vi "ProbePlanGenerator.vi"() -> ()   [LabVIEW 2013]
panel:
  in  "ATLAS 07 / ATLAS 12":u16(ring) items=["ATLAS 07", "ATLAS 12"]
  in  "innercut sensor?":bool
  in  "Filename":string="atlas12_innerc.txt"
  in  "Cancel Button":bool
  in  "Paste Button":bool
  in  "From 4-2":u16(ring) caption="From"
  in  "To 8":u16(ring) caption="To"
  in  "Column 4-2":u16(ring) caption="Column 2" items=["Column A", "Column B", "Column E", "Column C", "Column D"]
  in  "change4":bool caption="change columns?"
  in  "From 4-1":u16(ring) caption="From"
  in  "To 7":u16(ring) caption="To"
  in  "Column 4-1":u16(ring) caption="Column" items=["Column A", "Column B", "Column E", "Column C", "Column D"]
  in  "From 3-2":u16(ring) caption="From"
  in  "To 6":u16(ring) caption="To"
  in  "Column 3-2":u16(ring) caption="Column 2" items=["Column A", "Column B", "Column E", "Column C", "Column D"]
  in  "change3":bool caption="change columns?"
  in  "From 3-1":u16(ring) caption="From"
  in  "To 5":u16(ring) caption="To"
  in  "Column 3-1":u16(ring) caption="Column" items=["Column A", "Column B", "Column E", "Column C", "Column D"]
  in  "From 2-2":u16(ring) caption="From"
  in  "To 4":u16(ring) caption="To"
  in  "Column 2-2":u16(ring) caption="Column 2" items=["Column A", "Column B", "Column E", "Column C", "Column D"]
  in  "change2":bool caption="change columns?"
  in  "From 2-1":u16(ring) caption="From"
  in  "To 3":u16(ring) caption="To"
  in  "Column 2-1":u16(ring) caption="Column" items=["Column A", "Column B", "Column E", "Column C", "Column D"]
  in  "From 1-2":u16(ring) caption="From"
  in  "To 2":u16(ring) caption="To"
  in  "Column 1-2":u16(ring) caption="Column 2" items=["Column A", "Column B", "Column E", "Column C", "Column D"]
  in  "change1":bool caption="change columns?"
  in  "From 1-1":u16(ring) caption="From"
  in  "To":u16(ring)
  in  "Column 1-1":u16(ring) caption="Column" items=["Column A", "Column B", "Column E", "Column C", "Column D"]
  # "Probeplan Generator"
  # "Region 1"
  # "Region 2"
  # "Region 3"
  # "Region 4"
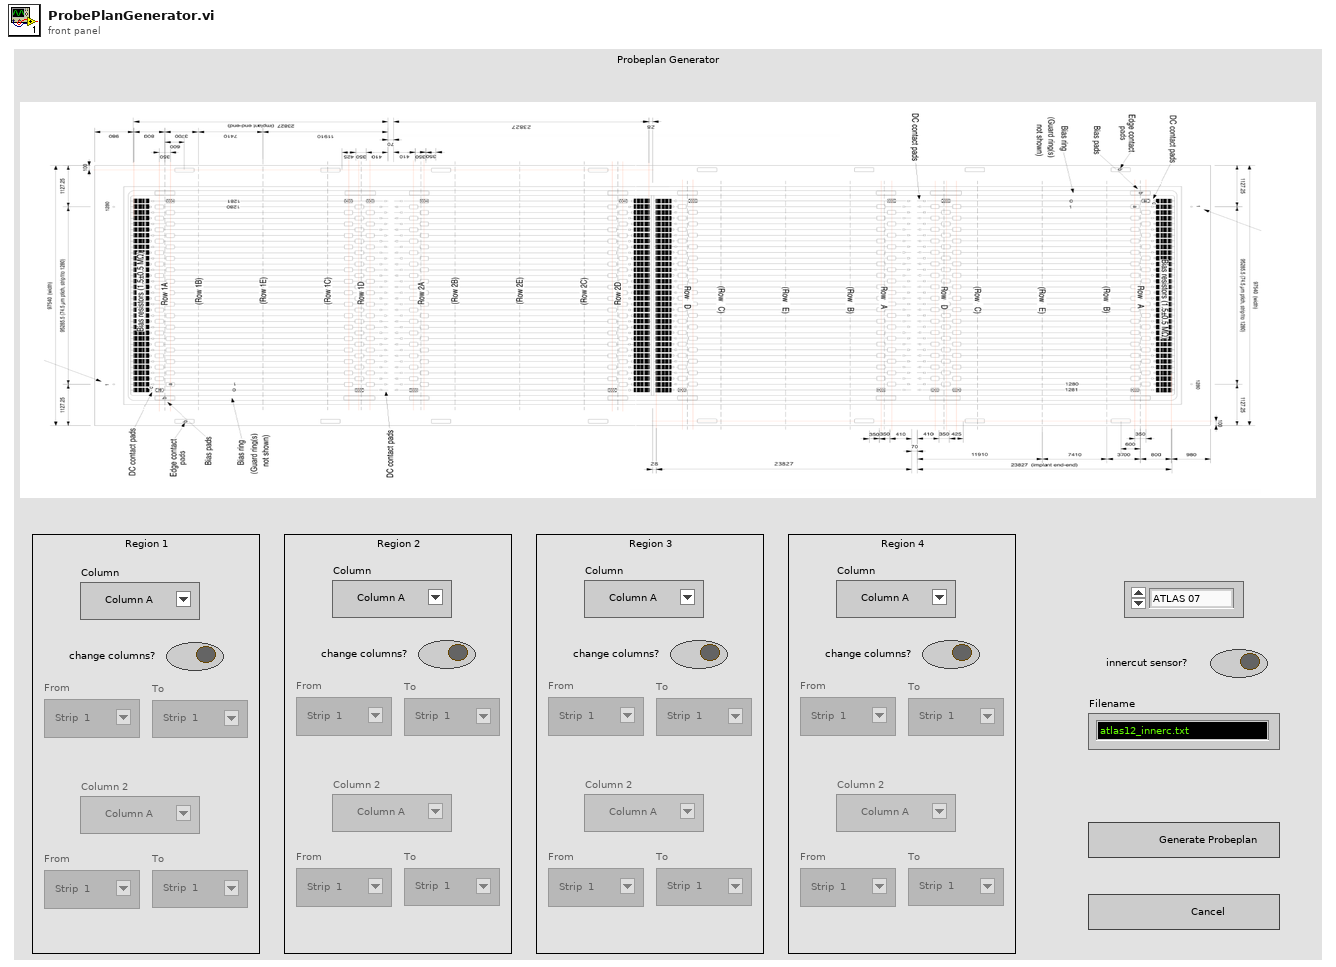
[diagram p1: front panel]
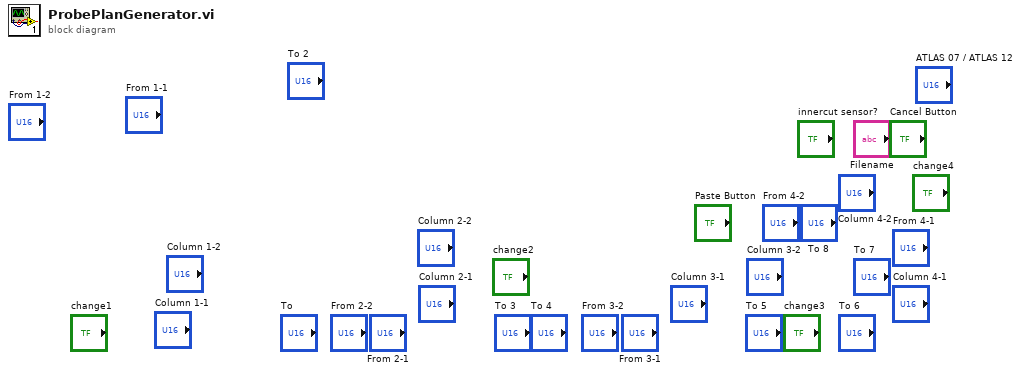
[diagram p0: block diagram]
diagram:
